vi "SpecialProcess.vi"(8 "error in":errorcluster caption="错误输入", 9 "Slot":T1, 10 "StrIn":string, 11 "N":i32) -> (0 "error out":errorcluster caption="错误输出", 3 "data":string)   [LabVIEW 2013]
uses:
  SystemCode/SysControl/Slot.ctl
  SourceCode/GlobalValue.vi
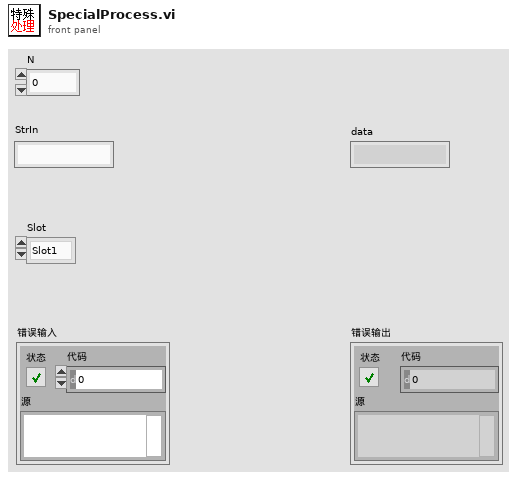
[diagram p1: front panel]
types:
  T1 = typedef "Slot.ctl" = enum16{"Slot1", "Slot2", "Slot3", "Slot4"}
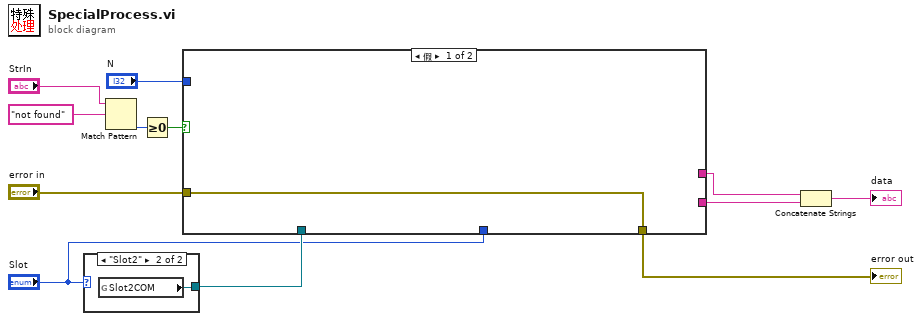
[diagram p0: block diagram]
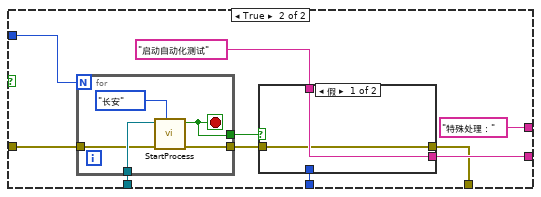
[diagram p2: hidden frame]
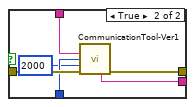
[diagram p3: hidden frame]
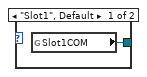
[diagram p4: hidden frame]
diagram:
  n1 = case shown="\"Slot2\"" "Slot" {
    tunnel: [w13 w14] -> w9
    frame "Slot1", Default {
      n2 = global read "GlobalValue.vi" "Slot1COM"() -> (w13:refnum<visa-resource-name>)
    }
    frame "Slot2" {
      n3 = global read "GlobalValue.vi" "Slot2COM"() -> (w14:refnum<visa-resource-name>)
    }
  }
  n4 = Match Pattern(string="StrIn", regular expression="not found") -> (offset past match=w10:i32)  [unwired: 1 in, 3 out]
  n5 = Greater Or Equal To 0?(x=w10) -> (x >= 0?=w8:bool)
  n6 = case shown="假" w8 {
    tunnel: w9 -> [_ w25]
    tunnel: "N" -> [_ w24]
    tunnel: "error in" -> [w15 w23]
    tunnel: "Slot" -> [_ w19]
    tunnel: [_ w18] -> w3
    tunnel: [w15 w17] -> w4
    tunnel: [_ "特殊处理：" ("字符串")] -> w1
    frame False {
    }
    frame True {
      n7 = for {
        N: w24 -> [_]
        tunnel: w25 -> [w38]
        tunnel: w23 -> [w36]
        tunnel: [w35] -> w22
        tunnel: [w34] -> w20
        stop <- w34 stop-if-true
        n8 = call "StartProcess.vi"("型号"=enum16{"长安", "江淮"}."长安", "error in"=w36, "COMIn"=w38) -> ("error out"=w35:errorcluster, "OK？"=w34:bool)  [unwired: 5 in, 2 out]
      }
      n9 = case shown="假" w20 {
        tunnel: w22 -> [w26 w33]
        tunnel: "启动自动化测试" ("通信协议名称") -> [w27 w32]
        tunnel: w19 -> [_ w31]
        tunnel: [w27 w29] -> w18
        tunnel: [w26 w28] -> w17
        frame False {
        }
        frame True {
          n10 = call "CommunicationTool-Ver1.vi"("通信协议名称"=w32, "Slot"=w31, "DelayTime"=u32 2000, "error in"=w33) -> ("data"=w29:string, "error out"=w28:errorcluster)  [unwired: 6 in, 4 out]
        }
      }
    }
  }
  "error out" <- w4
  n11 = Concatenate Strings(w1, w3) -> (→"data":string)
